vi "force_clamp_v3.vi"(2 "reinitialize? (F) 2":bool, 4 "handle in":i32, 6 "Pos 0":dbl, 7 "Desired Force (pN)":dbl, 8 "error in (no error)":errorcluster, 9 "QPD":dbl, 10 "Apply Force":bool, 11 "Nanostage":dbl) -> (0 "error out":errorcluster, 3 "QPD delta":dbl)   [LabVIEW 2026]
uses:
  <vilib>/addons/control/pid/pid.llb/PID (DBL).vi
  <vilib>/addons/control/pid/NI_PID_pid.lvlib
  Madlib.dll
panel:
  in  "dt (s)":dbl=-1.0 format="%.3f"
  out "Setpoint":dbl
  in  "output range":cluster{"output high":dbl, "output low":dbl}={"output high"=0.1, "output low"=-0.1} {"output low" format="%.2f"; "output high" format="%.2f"}
  out "PID output":dbl format="%.2f"
  in  "PID gains":T1={"proportional gain (Kc)"=0.5, "integral time (Ti, min)"=0.0, "derivative time (Td, min)"=0.0} {"derivative time (Td, min)" min=-1e-18 max=1000000000000000.0 step=1e-05 format="%.3f"; "integral time (Ti, min)" min=-1e-18 step=1e-05 format="%.6f"; "proportional gain (Kc)" min=-1e-18 step=1e-05 format="%.5f"}
  # "PID for holding a tethered DNA molecule ata constant force, determined by the BT value of the QPD.\nThe code is mainly inspired by the PID example VI shipped with LabVIEW. See it for further details."
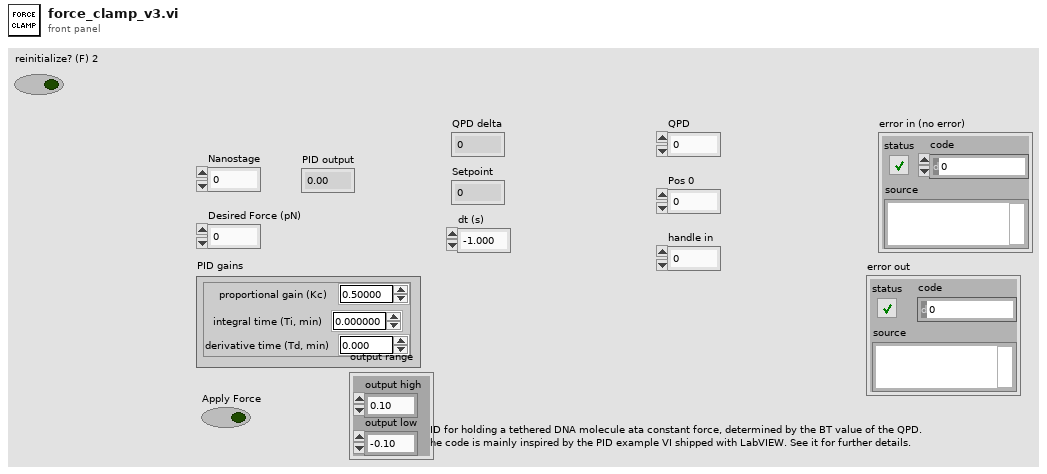
[diagram p1: front panel]
types:
  T1 = cluster{"proportional gain (Kc)":dbl, "integral time (Ti, min)":dbl, "derivative time (Td, min)":dbl}
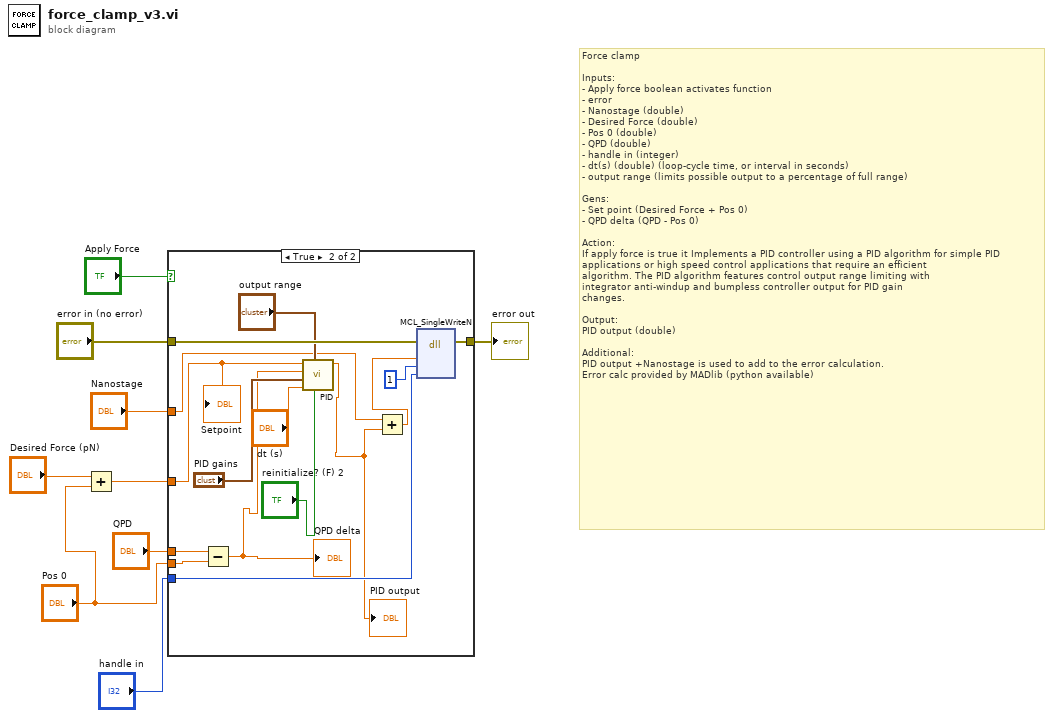
[diagram p0: block diagram]
diagram:
  # "Force clamp\n\nInputs:\n- Apply force boolean activates function\n- error\n- Nanostage (double)\n- Desired Force (double)\n- Pos 0 (double)\n- QPD (double)\n- handle in (integer)\n- dt(s) (double) (loop-cycle time, or interval in seconds)\n- output range (limits possible output to a percentage of full range)\n\nGens:\n- Set point (Desired Force + Pos 0)\n- QPD delta (QPD - Pos 0)\n\nAction:\nIf apply force is true it Implements a PID controller using a PID algorithm for simple PID \napplications or high speed control applications that require an efficient\nalgorithm. The PID algorithm features control output range limiting with\nintegrator anti-windup and bumpless controller output for PID gain \nchanges.\n\nOutput:\nPID output (double)\n\nAdditional:\nPID output +Nanostage is used to add to the error calculation.\nError calc provided by MADlib (python available)"
  n1 = Add(x="Desired Force (pN)", y="Pos 0") -> (x+y=w1:dbl)
  n2 = case shown="True" "Apply Force" {
    tunnel: "QPD" -> [_ w25]
    tunnel: "Pos 0" -> [_ w22]
    tunnel: w1 -> [_ w21]
    tunnel: "Nanostage" -> [_ w15]
    tunnel: "handle in" -> [_ w20]
    tunnel: "error in (no error)" -> [w10 w19]
    tunnel: [w10 w18] -> w4
    frame False {
    }
    frame True {
      n3 = Subtract(x=w25, y=w22) -> (x-y=w14:dbl)
      "QPD delta" <- w14
      n4 = call-poly <vilib>:"PID.vi"("reinitialize? (F)"="reinitialize? (F) 2", "output range"="output range", "dt (s)"="dt (s)", "PID gains"="PID gains", "process variable"=w14, "setpoint"=w21) -> ("output"=w12:dbl)  [unwired: 4 in, 1 out]
      "PID output" <- w12
      n5 = Add(x=w15, y=w12) -> (x+y=w16:dbl)
      n6 = dll-call lib="C:/Users/psmr500/PycharmProjects/COMBI-Tweez/LabVIEW Microscope Control/Nanostage/MADLib.dll" fn="MCL_SingleWriteN"(error in=w19, "position"=w16, "axis"=u32 1, "handle"=w20) -> (error out=w18:errorcluster)  [unwired: 6 in, 1 out]
      "Setpoint" <- w21
    }
  }
  "error out" <- w4
